vi "disconnectPubDataPublish.vi"(8 "error in (no error)":errorcluster, 11 "MiddlewareSVThisComponent in":refnum<class "MiddlewareSVThisComponent.lvclass">) -> (0 "error out":errorcluster, 3 "MiddlewareSVThisComponent out":refnum<class "MiddlewareSVThisComponent.lvclass">)   [LabVIEW 2015, in "MiddlewareSVThisComponent.lvclass"]
uses:
  MiddlewareSVThisComponent.lvclass
  MiddlewareSVThisComponent.lvclass/MiddlewareSVThisComponent.ctl
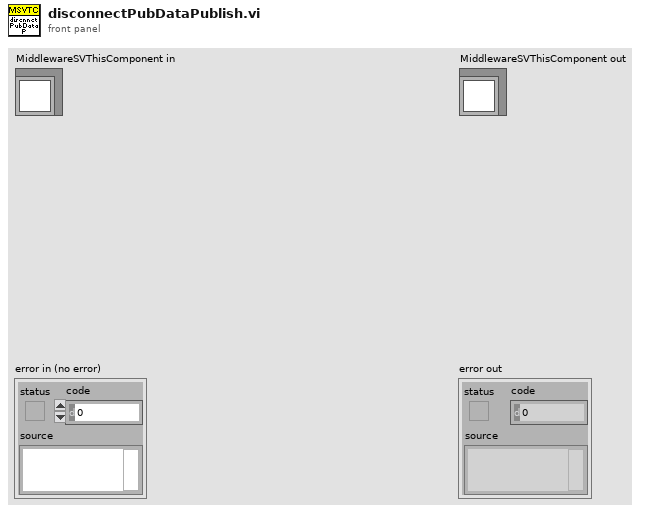
[diagram p1: front panel]
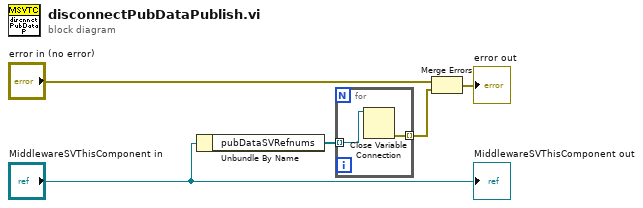
[diagram p0: block diagram]
diagram:
  n1 = Unbundle By Name("MiddlewareSVThisComponent in") -> ("pubDataSVRefnums"=w5:refnum<k21>[])
  n2 = for {
    tunnel: w5 -> [w7] mode=indexing
    tunnel: [w6] -> w3 mode=indexing
    n3 = Close Variable Connection(11:w7) -> (0:w6:errorcluster)  [unwired: 1 in]
  }
  n4 = Merge Errors("error in (no error)", w3) -> (→"error out":errorcluster)
  "MiddlewareSVThisComponent out" <- "MiddlewareSVThisComponent in"
